vi "PH_DeformableMirror.SetHV.vi"(0 "i ref in":refnum<vi>, 2 "HV on/off":bool, 5 "error in":errorcluster) -> (14 "i ref out":refnum<vi>, 19 "error out":errorcluster)   [LabVIEW 2014, in "PH_DeformableMirror.lvlib"]
uses:
  PH_DeformableMirror.lvlib
  instr.lib/dmdriver/DMirrorBase/DMirrorBase.lvclass
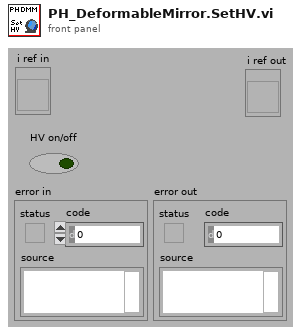
[diagram p1: front panel]
types:
  T1 = typedef "PH_DeformableMirror.lvlib/PH_DeformableMirror.i attribute.ctl" = cluster{"DMirror.lvlib:DMirrorBase.lvclass":refnum<class "DMirrorBase.lvclass">, "Device error":errorcluster, "GUI Refs":cluster{"Delete":refnum<vi>, "Device Error":refnum<vi>, "HV on":refnum<vi>, "Channel":refnum<vi>, "Voltage":refnum<vi>, "Channel Voltages":refnum<vi>}}
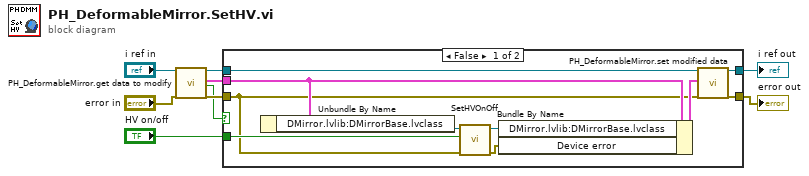
[diagram p0: block diagram]
diagram:
  n1 = call "PH_DeformableMirror.get data to modify.vi"("i ref in"="i ref in", "error in (no error)"="error in") -> ("i ref out"=w5:refnum<vi>, "i attribute"=w2:T1, "timed out"=w1:bool, "error out"=w3:errorcluster)  [unwired: 14 in]
  n2 = case shown="False" w1 {
    tunnel: [w19 w21] -> w9
    tunnel: "HV on/off" -> [w18 _]
    tunnel: w5 -> [w17 w21]
    tunnel: [w16 w20] -> w4
    tunnel: w3 -> [w10 w20]
    tunnel: w2 -> [w15 _]
    frame False {
      n3 = Unbundle By Name(w15) -> ("DMirror.lvlib:DMirrorBase.lvclass"=w14:refnum<class "DMirrorBase.lvclass">)
      n4 = call-dynamic "SetHVOnOff.vi"("error in (no error)"=w10, "HV On/Off"=w18, "DMirrorBase in"=w14) -> ("error out"=w11:errorcluster, "DMirrorBase out"=w12:refnum<class "DMirrorBase.lvclass">)  [unwired: 7 in]
      n5 = Bundle By Name(cluster=w15, "DMirror.lvlib:DMirrorBase.lvclass"=w12, "Device error"=w11) -> (w13:T1)
      n6 = call "PH_DeformableMirror.set modified data.vi"("i ref in"=w17, "i attribute"=w13, "error in (no error)"=w10) -> ("i ref out"=w19:refnum<vi>, "error out"=w16:errorcluster)  [unwired: 15 in]
    }
    frame True {
    }
  }
  "error out" <- w4
  "i ref out" <- w9
